vi "FestoCPX.getCPXerror.vi"(1 "CPX error":u8) -> (0 "CPX error explanation":string)   [LabVIEW 2013]
panel:
  # "out"
  # "in"
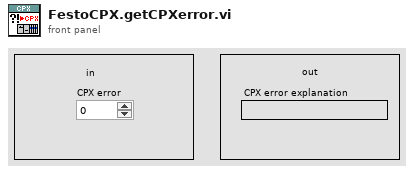
[diagram p1: front panel]
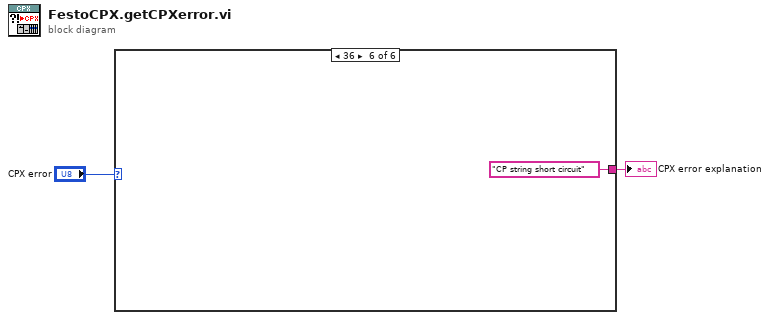
[diagram p0: block diagram]
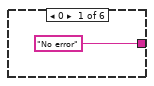
[diagram p2: hidden frame]
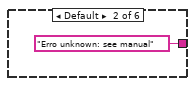
[diagram p3: hidden frame]
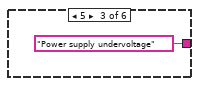
[diagram p4: hidden frame]
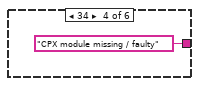
[diagram p5: hidden frame]
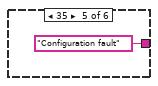
[diagram p6: hidden frame]
diagram:
  n1 = case shown="36" "CPX error" {
    tunnel: ["No error" "Erro unknown: see manual" "Power supply undervoltage" "CPX module missing / faulty" "Configuration fault" "CP string short circuit"] -> w1
    frame 0 {
    }
    frame Default {
    }
    frame 5 {
    }
    frame 34 {
    }
    frame 35 {
    }
    frame 36 {
    }
  }
  "CPX error explanation" <- w1
